vi "GetData&Date's.vi"(11 "file: (fromSite.txt)":path) -> (0 "asArray":dbl[][](array[numeric]), 2 "LRowAsArr":dbl[](array[numeric]) format="%#_2g", 3 "LastDate":string)   [LabVIEW 2023]
uses:
  <vilib>/Utility/file.llb/Read Delimited Spreadsheet (string).vi
panel:
  out "LTxtLine":string
  out "size(s)":i32
  out "asString":string[](array[string])
  out "All rows":string[][](array[string])
  out "From File":string
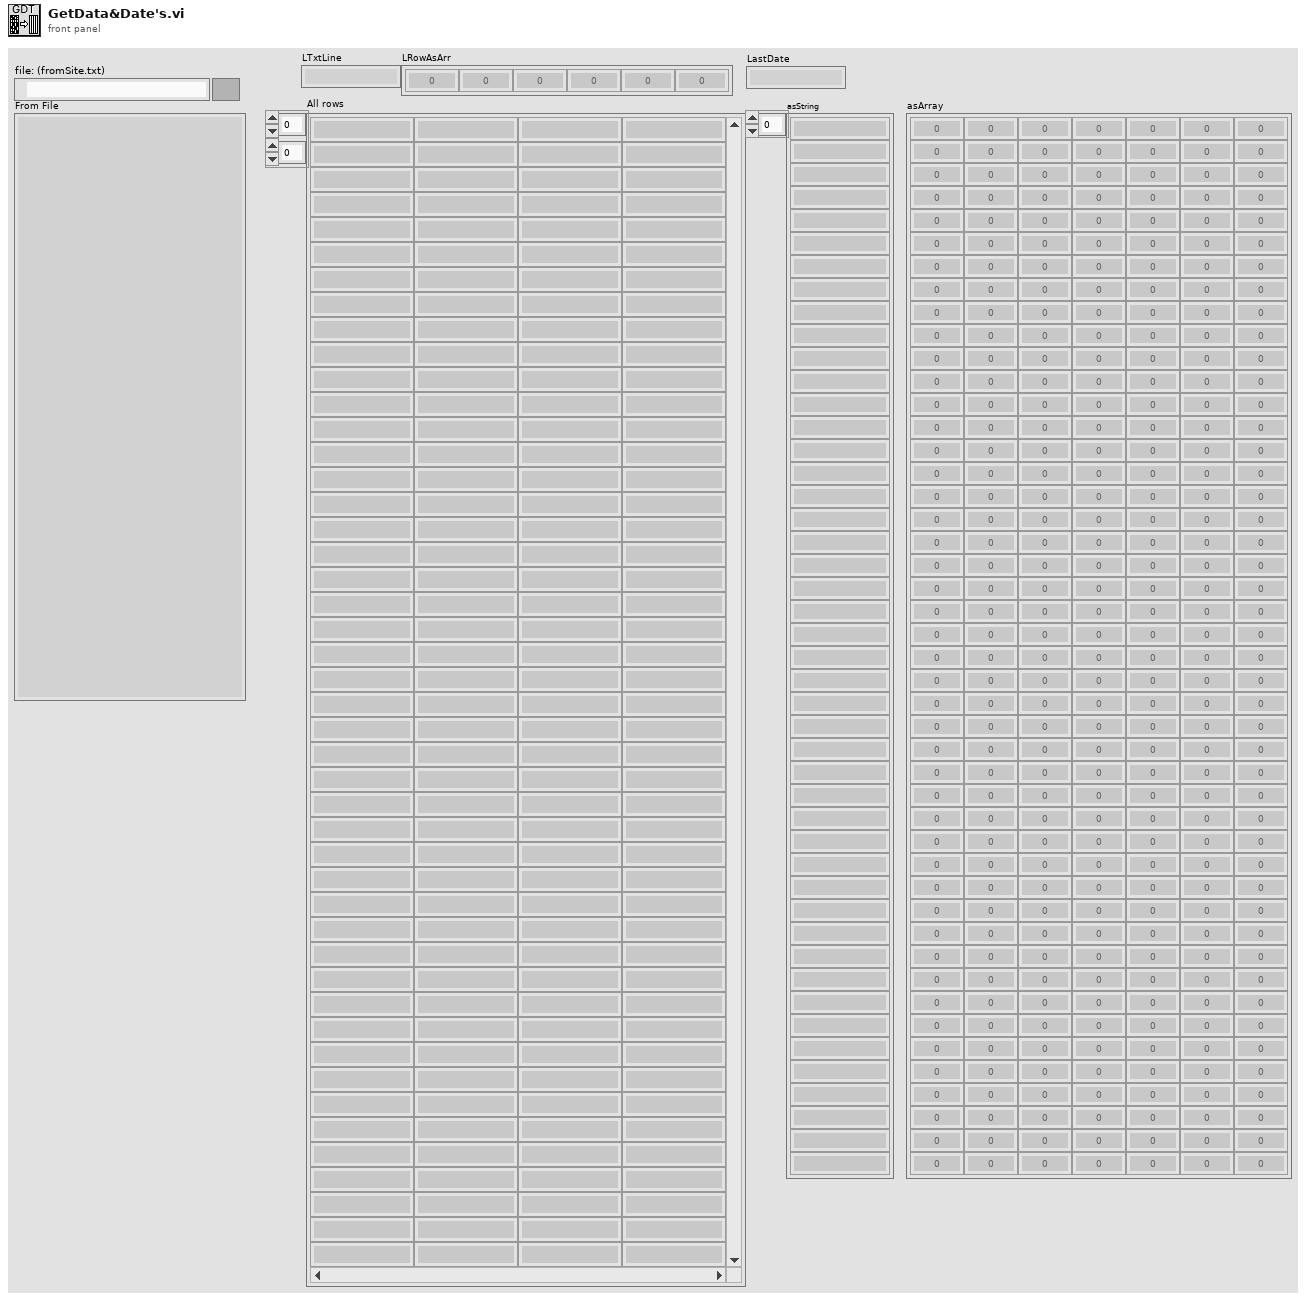
[diagram p1: front panel]
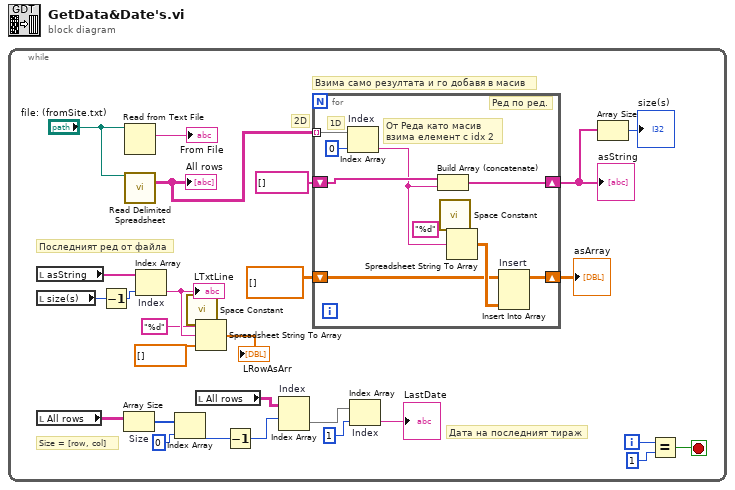
[diagram p0: block diagram]
diagram:
  n1 = while {
    i -> [w3]
    stop <- w2 stop-if-true
    # "Size = [row, col]"
    # "2D"
    # "Последният ред от файла"
    # "Дата на последният тираж"
    # "Взима само резултата и го добавя в масив"
    n2 = local read "asString"() -> (w23:string[])
    n3 = local read "size(s)"() -> (w22:i32)
    n4 = local read "All rows"() -> (w9:string[][])
    n5 = Decrement(x=w22) -> (x-1=w21:i32)
    n6 = Array Size "Size"(array=w9) -> (size(s)=w12:i32[])
    n7 = Read from Text File(file (use dialog)="file: (fromSite.txt)") -> (text=→"From File":string)  [unwired: 3 in, 3 out]
    n8 = call-poly <vilib>:"Read Delimited Spreadsheet.vi"("file path (dialog if empty)"="file: (fromSite.txt)") -> ("all rows"=w26:string[][])  [unwired: 9 in, 5 out]
    "All rows" <- w26
    n9 = Index Array "Index"(array=w23, index=w21) -> (element=w17:string)
    "LTxtLine" <- w17
    n10 = Index Array(array=w12, index=0) -> (element=w10:i32)
    n11 = call <vilib>:"Space Constant.vi"() -> ("String"=w15:string)
    n12 = Spreadsheet String To Array(delimiter (Tab)=w15, format string="%d", spreadsheet string=w17, array type (2D Dbl)=dbl[] []) -> (array=→"LRowAsArr":dbl[])
    n13 = local read "All rows"() -> (w4:string[][])
    n14 = Decrement(x=w10) -> (x-1=w8:i32)
    n15 = Index Array "Index"(array=w4, index (row)=w8) -> (element=w7:string[])  [unwired: 1 in]
    n16 = for {
      tunnel: w26 -> [w38] mode=indexing
      shift-right: [w36] -> w20
      shift-left: string[] [] -> [w35]
      shift-right: [w30] -> w18
      shift-left: dbl[][] [] -> [w29]
      # "От Реда като масив \nвзима елемент с idx 2"
      # "1D"
      # "Ред по ред."
      n17 = Index Array "Index"(array=w38, index=0) -> (element=w34:string)
      n18 = Build Array (concatenate)(w35, w34) -> (w36:string[])
      n19 = call <vilib>:"Space Constant.vi"() -> ("String"=w32:string)
      n20 = Spreadsheet String To Array(delimiter (Tab)=w32, format string="%d", spreadsheet string=w34) -> (array=w31:dbl[][])  [unwired: 1 in]
      n21 = Insert Into Array "Insert"(array=w29, new element=w31) -> (w30:dbl[][])  [unwired: 2 in]
    }
    "asString" <- w20
    "asArray" <- w18
    n22 = Index Array "Index"(array=w7, index=1) -> (element=→"LastDate":string)
    n23 = Array Size(array=w20) -> (size(s)=→"size(s)":i32)
    n24 = Equal?(x=w3, y=1) -> (x = y?=w2:bool)
  }
